vi "Parse User Role.vi"(8 "error in (no error)":errorcluster, 11 "role":string) -> (0 "error out":errorcluster, 3 "Role":T1)   [LabVIEW 2026, in "Local File Auth Provider.lvclass"]
uses:
  Local File Auth Provider.lvclass
  Local File Auth Provider.lvclass/Local File Auth Provider.ctl
  Typedefs/enums/Role Enum.ctl
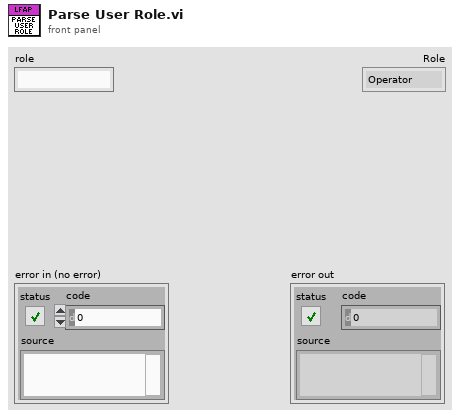
[diagram p1: front panel]
types:
  T1 = typedef "Role Enum.ctl" = enum16{"Operator", "Engineer", "Admin"}
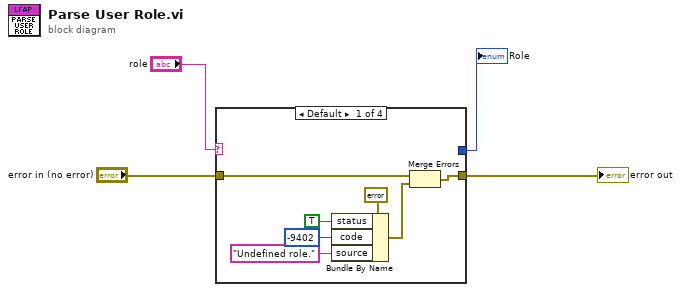
[diagram p0: block diagram]
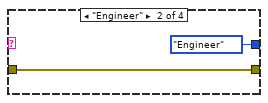
[diagram p2: hidden frame]
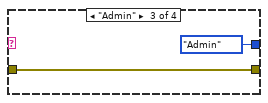
[diagram p3: hidden frame]
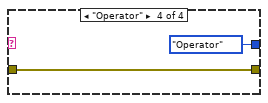
[diagram p4: hidden frame]
diagram:
  n1 = case shown="Default" "role" {
    tunnel: [_ Role_Enum."Engineer" ("Role") Role_Enum."Admin" ("Role") Role_Enum."Operator" ("Role")] -> w4
    tunnel: "error in (no error)" -> [w7 w13 w15 w17]
    tunnel: [w5 w13 w15 w17] -> w3
    frame Default {
      n2 = Bundle By Name(cluster=errorcluster {"status"=FALSE, "code"=0, "source"=""} ("error out"), "status"=TRUE, "code"=-9402, "source"="Undefined role.") -> (w6:errorcluster)
      n3 = Merge Errors(w7, w6) -> (w5:errorcluster)
    }
    frame "Engineer" {
    }
    frame "Admin" {
    }
    frame "Operator" {
    }
  }
  "Role" <- w4
  "error out" <- w3
